vi "Find Annotation Times.vi"(8 "error in":errorcluster, 11 "Full Text String Array":string[][](array[string])) -> (0 "error out":errorcluster, 1 "End Times":dbl[](array[numeric]), 2 "Start Times":dbl[](array[numeric]), 3 "Event Names":string[](array[string]), 4 "Event Times":dbl[](array[numeric]), 5 "Has Annotations?":bool)   [LabVIEW 2021]
panel:
  out "Annotation Table":string[][](table)
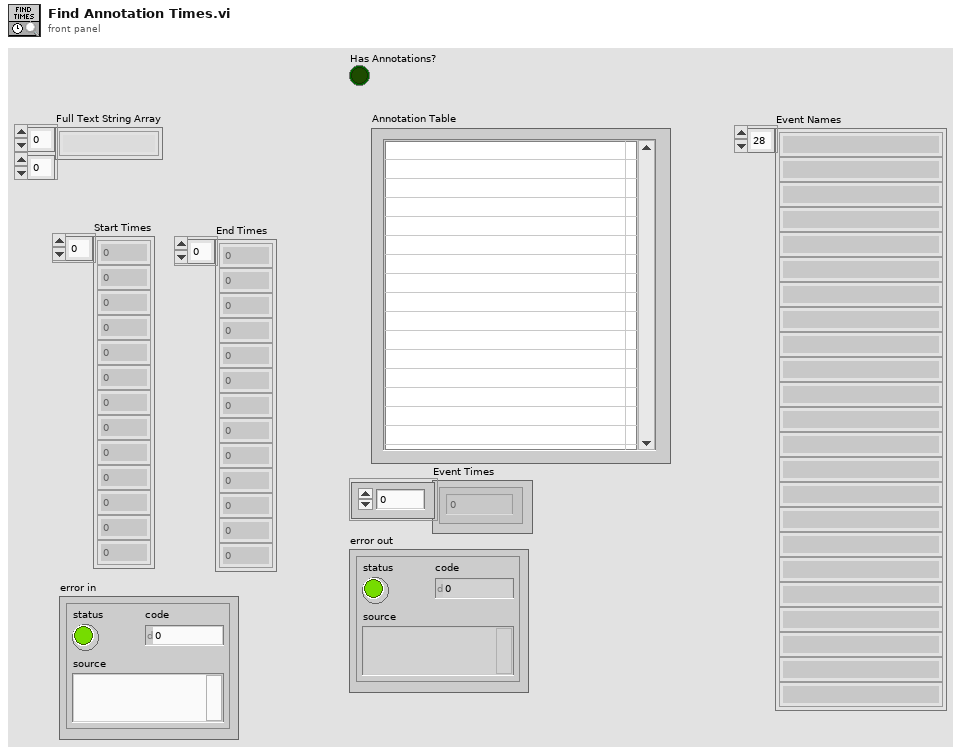
[diagram p1: front panel]
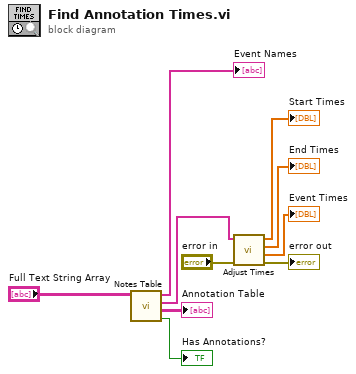
[diagram p0: block diagram]
diagram:
  n1 = call "Notes Table.vi"("Full Text String Array"="Full Text String Array") -> ("Has Annotations?"=→"Has Annotations?":bool, "Annotation Table"=→"Annotation Table":string[][], "Times"=w6:string[], "Labels"=→"Event Names":string[])  [unwired: 7 in]
  n2 = call "Adjust Times.vi"("error in"="error in", "Times"=w6) -> ("error out"=→"error out":errorcluster, "Event Times"=→"Event Times":dbl[], "End Times"=→"End Times":dbl[], "Start Times"=→"Start Times":dbl[])  [unwired: 6 in]
